vi "FL Function Interpolation.vi"(6 "user-defined \nshape index":i32, 7 "user MF interpolating polynomials":T1[](array[typedef]) {"coa_x(y) coeff" format="%.4g"; "Area(y) coeff" format="%.4g"; "X(y) coeff" format="%.4g"; "Y(x) coeff" format="%.4g"; "Y" format="%.4g"; "X" format="%.4g"}, 9 "Input Data":dbl, 10 "shape":T2 items=["Triangle", "Trapezoid", "Singleton", "Sigmoid", "Gaussian", "User-Defined"], 11 "Points":dbl[](array[numeric])=[0.0, 0.0, 0.0, 0.0]) -> (1 "Membership":dbl)   [LabVIEW 2020, in "NI_Fuzzy_Logic_API.lvlib"]
uses:
  <vilib>/addons/Fuzzy Logic/NI_Fuzzy_Logic_API.lvlib
  <vilib>/addons/Fuzzy Logic/TypeDefs/FL Membership Function Shape.ctl
  <vilib>/addons/Fuzzy Logic/TypeDefs/FL Interpolating polynomials.ctl
panel:
  # "This VI calculates the Membership, by using Points to create rising and falling arrays, and then a linear\nor cubic interpolation is used, depending on Function.\n\nSigm = f(x) = 1 / (1+e^(-x))\n\nGaussian = f(x) =1*e^(-1(x-0)^2)"
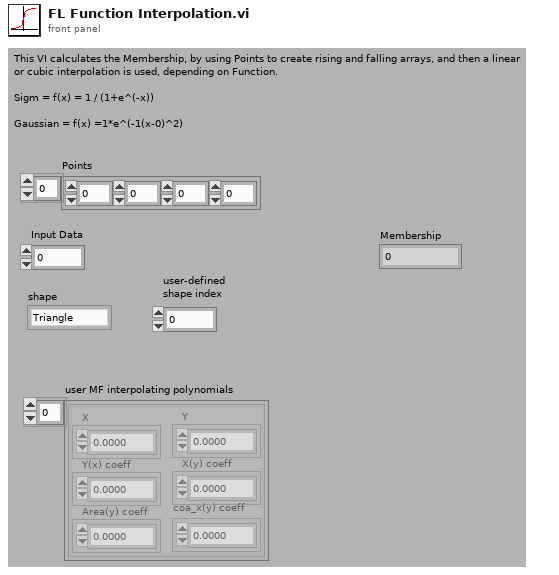
[diagram p1: front panel]
types:
  T1 = typedef "NI_Fuzzy_Logic_API.lvlib/FL Interpolating polynomials.ctl" = cluster{"X":dbl[], "Y":dbl[], "Y(x) coeff":dbl[][], "X(y) coeff":dbl[][], "Area(y) coeff":dbl[][], "coa_x(y) coeff":dbl[][]}
  T2 = typedef "NI_Fuzzy_Logic_API.lvlib/FL Membership Function Shape.ctl" = u16
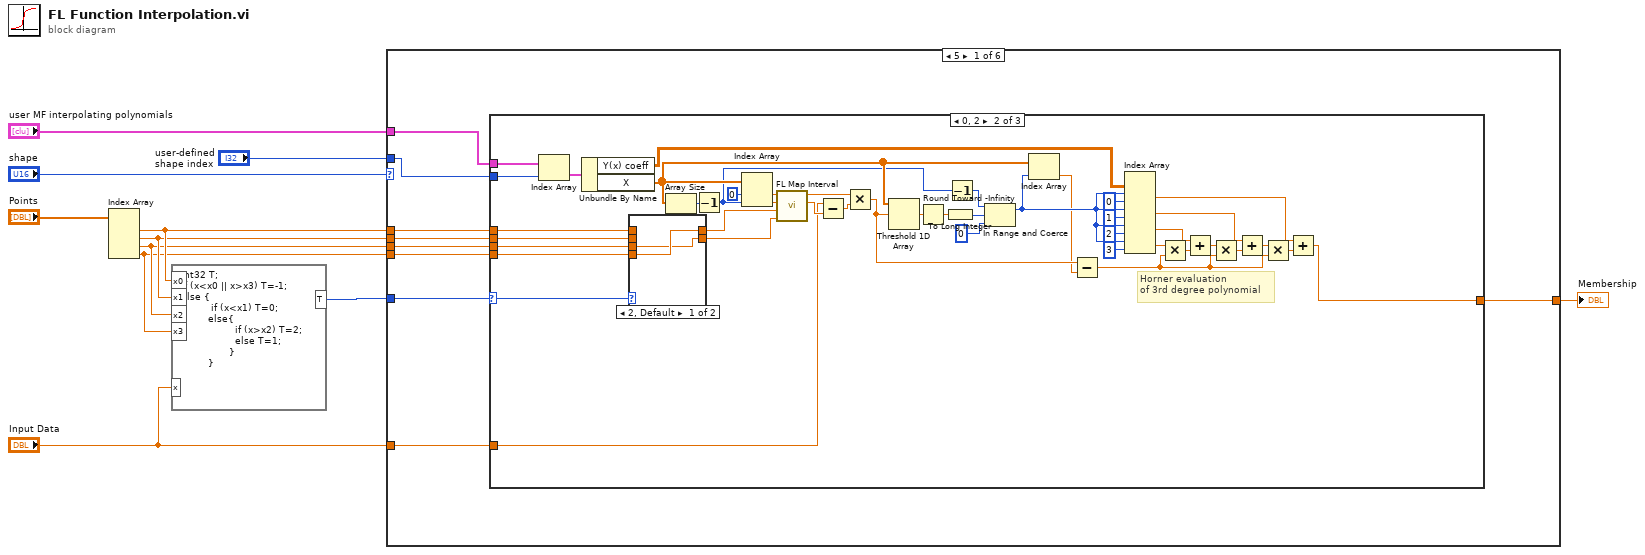
[diagram p0: block diagram]
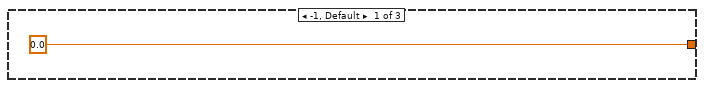
[diagram p2: hidden frame]
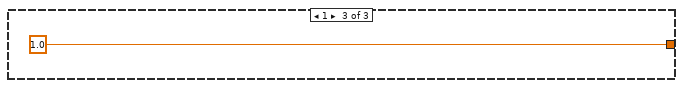
[diagram p4: hidden frame]
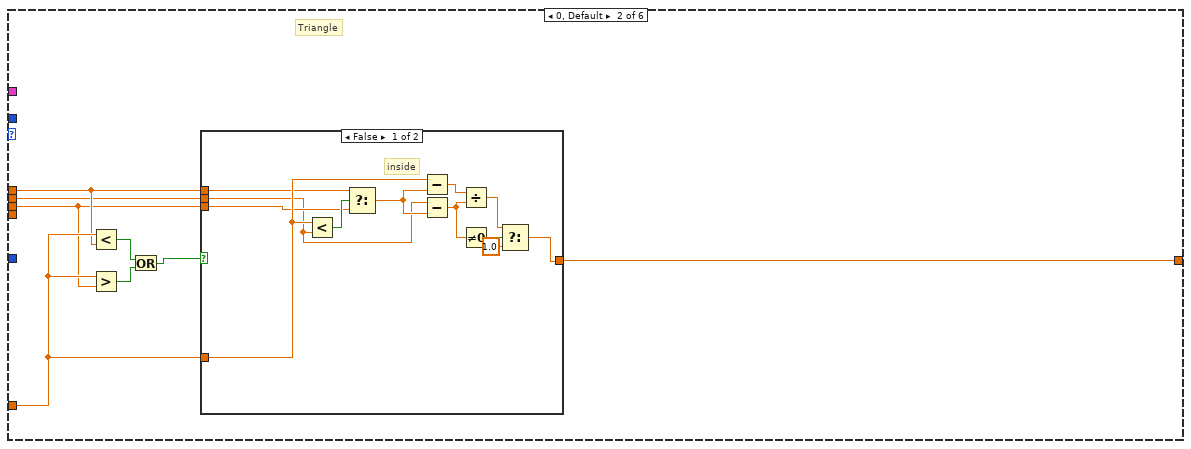
[diagram p5: hidden frame]
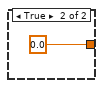
[diagram p6: hidden frame]
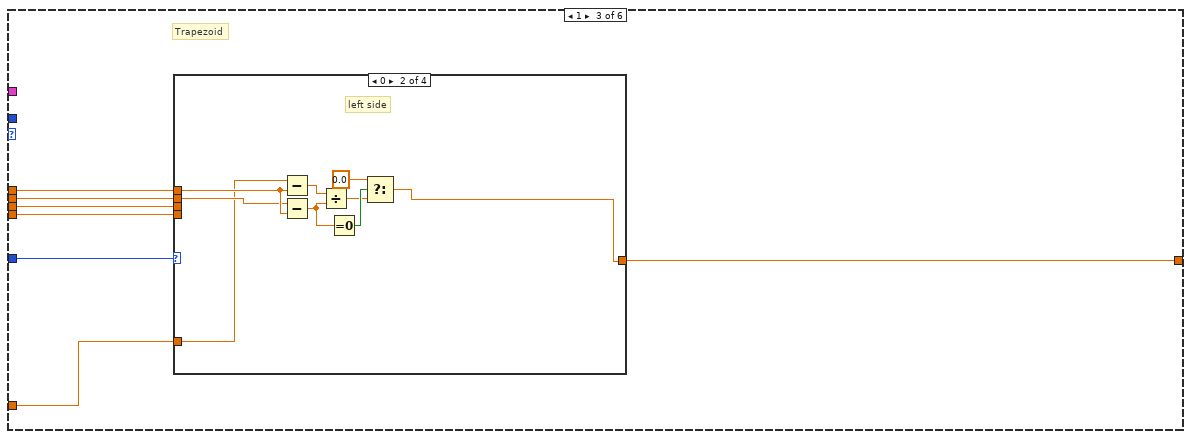
[diagram p7: hidden frame]
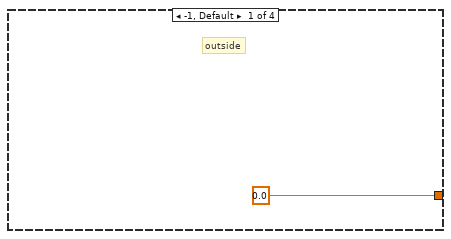
[diagram p8: hidden frame]
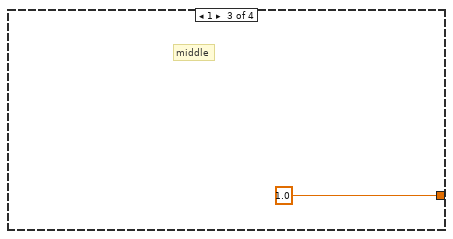
[diagram p9: hidden frame]
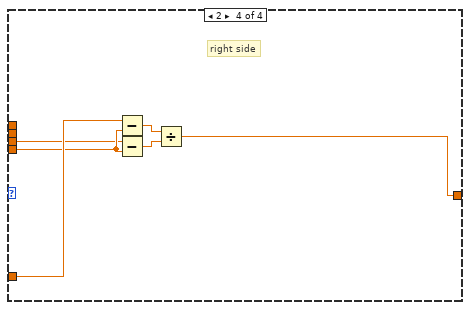
[diagram p10: hidden frame]
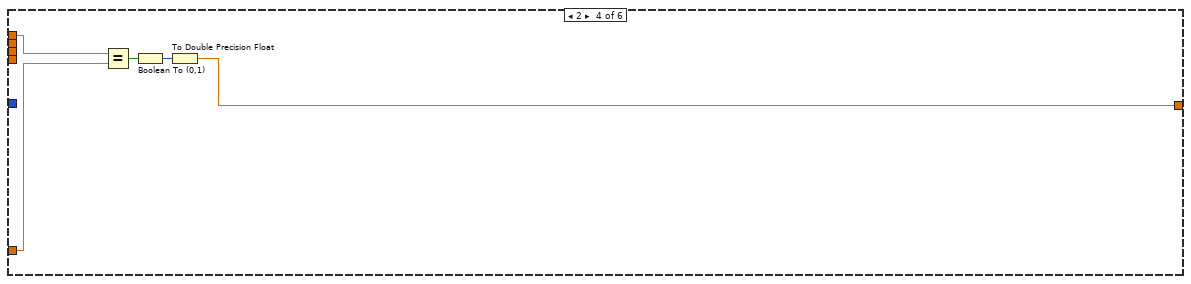
[diagram p11: hidden frame]
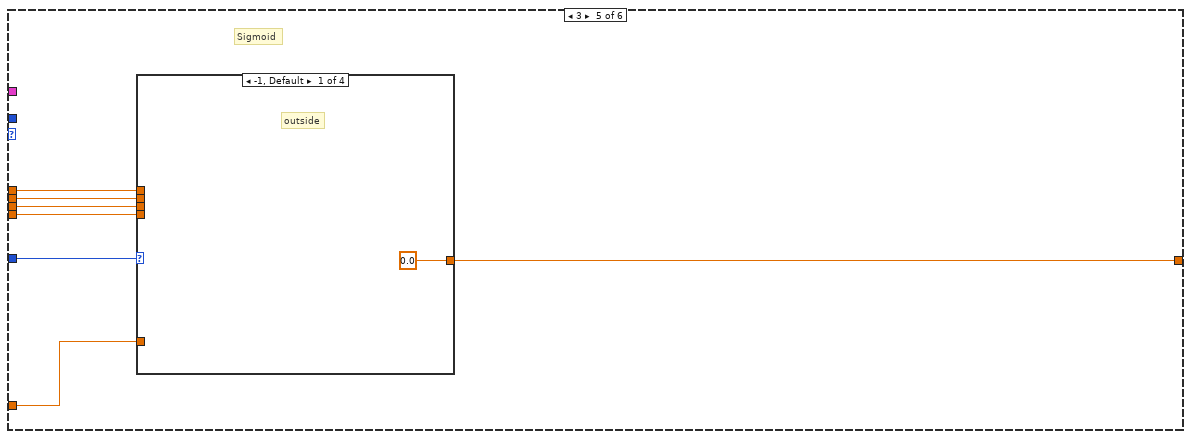
[diagram p12: hidden frame]
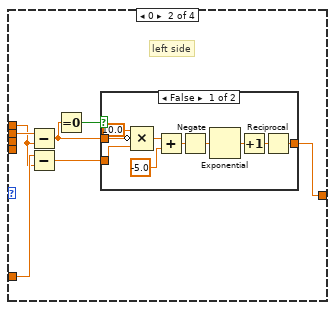
[diagram p13: hidden frame]
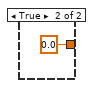
[diagram p14: hidden frame]
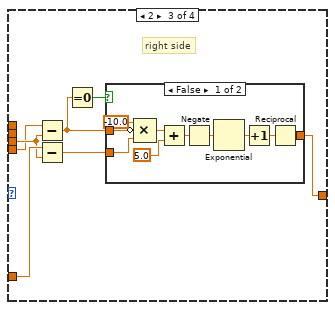
[diagram p15: hidden frame]
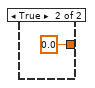
[diagram p16: hidden frame]
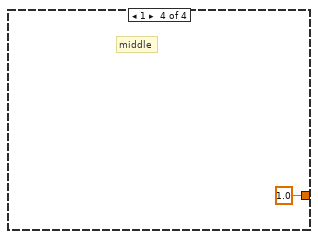
[diagram p17: hidden frame]
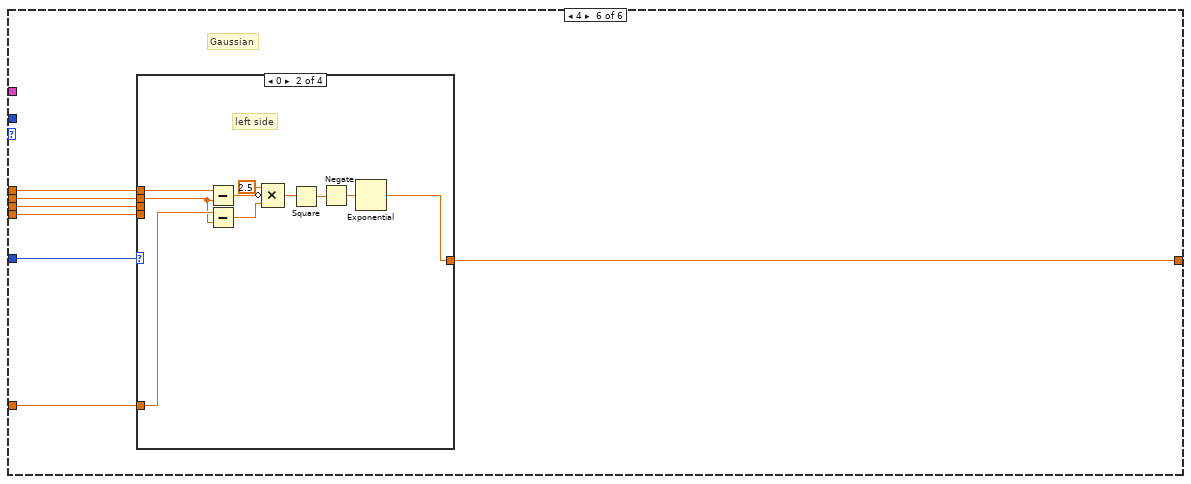
[diagram p18: hidden frame]
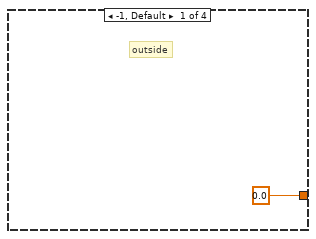
[diagram p19: hidden frame]
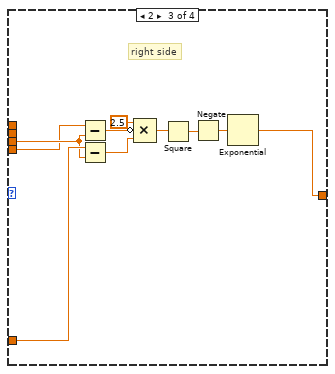
[diagram p20: hidden frame]
diagram:
  n1 = Index Array(array="Points") -> (element #1=w8:dbl, element #2=w7:dbl, element #3=w6:dbl, element #4=w5:dbl)  [unwired: 4 in]
  n2 = formula code="int32 T;\nif (x<x0 || x>x3) T=-1;\nelse {\n          if (x<x1) T=0;\n         else{\n                  if (x>x2) T=2;\n                  else T=1;\n                }\n         }"("x0"=w8, "x1"=w7, "x2"=w6, "x3"=w5, "x"="Input Data") -> ("T"=w3:i32)
  n3 = case shown="5" "shape" {
    tunnel: "Input Data" -> [w19 w78 w98 w119 w127 w172]
    tunnel: [w20 w77 w97 w116 w126 w171] -> w10
    tunnel: w8 -> [w18 w76 w96 w120 w124 w170]
    tunnel: w7 -> [w17 w75 w95 _ w123 w169]
    tunnel: w6 -> [w16 w74 w94 _ w122 w168]
    tunnel: w5 -> [w15 _ w93 _ w121 w167]
    tunnel: w3 -> [w14 _ w92 _ w125 w166]
    tunnel: "user MF interpolating polynomials" -> [w13 _ _ _ _ _]
    tunnel: "user-defined \nshape index" -> [w12 _ _ _ _ _]
    frame 5 {
      n4 = case shown="0, 2" w14 {
        selector: w14 -> [_ w31 _]
        tunnel: [0.0 w57 1.0] -> w20
        tunnel: w18 -> [_ w30 _]
        tunnel: w17 -> [_ w29 _]
        tunnel: w16 -> [_ w28 _]
        tunnel: w15 -> [_ w27 _]
        tunnel: w19 -> [_ w61 _]
        tunnel: w13 -> [_ w23 _]
        tunnel: w12 -> [_ w22 _]
        frame -1, Default {
        }
        frame 0, 2 {
          # "Horner evaluation\nof 3rd degree polynomial"
          n5 = Index Array(array=w23, index=w22) -> (element=w24:T1)
          n6 = Unbundle By Name(w24) -> ("Y(x) coeff"=w35:dbl[][], "X"=w36:dbl[])
          n7 = case shown="2, Default" w31 {
            tunnel: w30 -> [_ w69]
            tunnel: w29 -> [_ w68]
            tunnel: w28 -> [w66 _]
            tunnel: w27 -> [w67 _]
            tunnel: [w67 w69] -> w26
            tunnel: [w66 w68] -> w25
            frame 2, Default {
            }
            frame 0 {
            }
          }
          n8 = Array Size(array=w36) -> (size(s)=w34:i32)
          n9 = Decrement(x=w34) -> (x-1=w33:i32)
          n10 = Index Array(array=w36, index #1=0 ("index"), index #2=w33) -> (element #1=w64:dbl, element #2=w63:dbl)
          n11 = call <vilib>:"FL Map Interval.vi"("x1"=w25, "x0"=w26, "b"=w63, "a"=w64) -> ("m"=w62:dbl, "k"=w60:dbl)  [unwired: 6 out]
          n12 = Subtract(x=w61, y=w62) -> (x-y=w59:dbl)
          n13 = Multiply(x=w60, y=w59) -> (x*y=w58:dbl)
          n14 = Threshold 1D Array(2:w58, 3:w36) -> (0:w38:dbl)  [unwired: 1 out]
          n15 = Round Toward -Infinity(1:w38) -> (0:w39:dbl)
          n16 = To Long Integer(number=w39) -> (32bit integer=w40:i32)
          n17 = Decrement(x=w33) -> (x-1=w32:i32)
          n18 = In Range and Coerce(upper limit=w32, x=w40, lower limit=0) -> (coerced(x)=w42:i32)  [unwired: 1 out]
          n19 = Index Array(array=w36, index=w42) -> (element=w37:dbl)
          n20 = Subtract(x=w58, y=w37) -> (x-y=w54:dbl)
          n21 = Index Array(array=w35, index (row) #1=w42, index (col) #1=0 ("disabled index (col)"), index (row) #2=w42, index (col) #2=1 ("disabled index (col)"), index (row) #3=w42, index (col) #3=2 ("disabled index (col)"), index (row) #4=w42, index (col) #4=3 ("disabled index (col)")) -> (element #1=w56:dbl, element #2=w52:dbl, element #3=w49:dbl, element #4=w47:dbl)
          n22 = Multiply(x=w47, y=w54) -> (x*y=w48:dbl)
          n23 = Add(x=w49, y=w48) -> (x+y=w50:dbl)
          n24 = Multiply(x=w50, y=w54) -> (x*y=w51:dbl)
          n25 = Add(x=w52, y=w51) -> (x+y=w53:dbl)
          n26 = Multiply(x=w53, y=w54) -> (x*y=w55:dbl)
          n27 = Add(x=w56, y=w55) -> (x+y=w57:dbl)
        }
        frame 1 {
        }
      }
    }
    frame 0, Default {
      # "Triangle"
      n28 = Less?(x=w78, y=w76) -> (x < y?=w73:bool)
      n29 = Greater?(x=w78, y=w74) -> (0:w72:bool)
      n30 = Or(x=w73, y=w72) -> (x .or. y?=w71:bool)
      n31 = case shown="False" w71 {
        tunnel: [w79 0.0 ("Membership")] -> w77
        tunnel: w76 -> [w86 _]
        tunnel: w75 -> [w84 _]
        tunnel: w74 -> [w85 _]
        tunnel: w78 -> [w87 _]
        frame False {
          # "inside"
          n32 = Less?(x=w87, y=w84) -> (x < y?=w88:bool)
          n33 = Select(t=w86, s=w88, f=w85) -> (s? t:f=w89:dbl)
          n34 = Subtract(x=w87, y=w89) -> (x-y=w90:dbl)
          n35 = Subtract(x=w84, y=w89) -> (x-y=w83:dbl)
          n36 = Divide(x=w90, y=w83) -> (x/y=w80:dbl)
          n37 = Not Equal To 0?(x=w83) -> (x != 0?=w82:bool)
          n38 = Select(t=w80, s=w82, f=1.0) -> (s? t:f=w79:dbl)
        }
        frame True {
        }
      }
    }
    frame 1 {
      # "Trapezoid"
      n39 = case shown="0" w92 {
        tunnel: [0.0 w101 1.0 w110] -> w97
        tunnel: w96 -> [_ w107 _ _]
        tunnel: w95 -> [_ w106 _ _]
        tunnel: w94 -> [_ _ _ w112]
        tunnel: w93 -> [_ _ _ w113]
        tunnel: w98 -> [_ w105 _ w114]
        frame -1, Default {
          # "outside"
        }
        frame 0 {
          # "left side"
          n40 = Subtract(x=w105, y=w107) -> (x-y=w108:dbl)
          n41 = Subtract(x=w106, y=w107) -> (x-y=w100:dbl)
          n42 = Divide(x=w108, y=w100) -> (x/y=w102:dbl)
          n43 = Equal To 0?(x=w100) -> (x = 0?=w104:bool)
          n44 = Select(t=0.0, s=w104, f=w102) -> (s? t:f=w101:dbl)
        }
        frame 1 {
          # "middle"
        }
        frame 2 {
          # "right side"
          n45 = Subtract(x=w114, y=w113) -> (x-y=w115:dbl)
          n46 = Subtract(x=w112, y=w113) -> (x-y=w111:dbl)
          n47 = Divide(x=w115, y=w111) -> (x/y=w110:dbl)
        }
      }
    }
    frame 2 {
      n48 = Equal?(x=w120, y=w119) -> (x = y?=w118:bool)
      n49 = Boolean To (0,1)(Boolean=w118) -> (0, 1=w117:i16)
      n50 = To Double Precision Float(number=w117) -> (double precision float=w116:dbl)
    }
    frame 3 {
      # "Sigmoid"
      n51 = case shown="-1, Default" w125 {
        tunnel: [0.0 w133 w149 1.0] -> w126
        tunnel: w124 -> [_ w132 _ _]
        tunnel: w123 -> [_ w134 _ _]
        tunnel: w122 -> [_ _ w151 _]
        tunnel: w121 -> [_ _ w150 _]
        tunnel: w127 -> [_ w135 w153 _]
        frame -1, Default {
          # "outside"
        }
        frame 0 {
          # "left side"
          n52 = Subtract(x=w134, y=w132) -> (x-y=w129:dbl)
          n53 = Subtract(x=w135, y=w132) -> (x-y=w131:dbl)
          n54 = Equal To 0?(x=w129) -> (x = 0?=w130:bool)
          n55 = case shown="False" w130 {
            tunnel: w129 -> [w145 _]
            tunnel: [w139 0.0] -> w133
            tunnel: w131 -> [w136 _]
            frame False {
              n56 = Compound Arithmetic op=MULTIPLY(10.0 ("value"), invert w145, w136) -> (w141:dbl)
              n57 = Add(x=w141, y=-5.0) -> (x+y=w138:dbl)
              n58 = Negate(x=w138) -> (-x=w143:dbl)
              n59 = Exponential(1:w143) -> (0:w142:dbl)
              n60 = Increment(x=w142) -> (x+1=w140:dbl)
              n61 = Reciprocal(x=w140) -> (1/x=w139:dbl)
            }
            frame True {
            }
          }
        }
        frame 2 {
          # "right side"
          n62 = Subtract(x=w150, y=w151) -> (x-y=w148:dbl)
          n63 = Subtract(x=w153, y=w151) -> (x-y=w152:dbl)
          n64 = Equal To 0?(x=w148) -> (x = 0?=w147:bool)
          n65 = case shown="False" w147 {
            tunnel: w152 -> [w162 _]
            tunnel: [w157 0.0] -> w149
            tunnel: w148 -> [w154 _]
            frame False {
              n66 = Compound Arithmetic op=MULTIPLY(-10.0 ("value"), invert w154, w162) -> (w159:dbl)
              n67 = Add(x=w159, y=5.0) -> (x+y=w156:dbl)
              n68 = Negate(x=w156) -> (-x=w161:dbl)
              n69 = Exponential(1:w161) -> (0:w160:dbl)
              n70 = Increment(x=w160) -> (x+1=w158:dbl)
              n71 = Reciprocal(x=w158) -> (1/x=w157:dbl)
            }
            frame True {
            }
          }
        }
        frame 1 {
          # "middle"
        }
      }
    }
    frame 4 {
      # "Gaussian"
      n72 = case shown="0" w166 {
        tunnel: [0.0 w180 w192 1.0] -> w171
        tunnel: w170 -> [_ w182 _ _]
        tunnel: w169 -> [_ w181 _ _]
        tunnel: w168 -> [_ _ w191 _]
        tunnel: w167 -> [_ _ w190 _]
        tunnel: w172 -> [_ w183 w193 _]
        frame -1, Default {
          # "outside"
        }
        frame 0 {
          # "left side"
          n73 = Subtract(x=w182, y=w181) -> (x-y=w179:dbl)
          n74 = Subtract(x=w183, y=w181) -> (x-y=w177:dbl)
          n75 = Compound Arithmetic op=MULTIPLY(2.5 ("value"), invert w179, w177) -> (w176:dbl)
          n76 = Square(x=w176) -> (x^2=w175:dbl)
          n77 = Negate(x=w175) -> (-x=w174:dbl)
          n78 = Exponential(1:w174) -> (0:w180:dbl)
        }
        frame 2 {
          # "right side"
          n79 = Subtract(x=w190, y=w191) -> (x-y=w189:dbl)
          n80 = Subtract(x=w193, y=w191) -> (x-y=w187:dbl)
          n81 = Compound Arithmetic op=MULTIPLY(2.5 ("value"), invert w189, w187) -> (w186:dbl)
          n82 = Square(x=w186) -> (x^2=w185:dbl)
          n83 = Negate(x=w185) -> (-x=w184:dbl)
          n84 = Exponential(1:w184) -> (0:w192:dbl)
        }
        frame 1 {
          # "middle"
        }
      }
    }
  }
  "Membership" <- w10
